vi "Hintergrund durchfuehren FT-IR.vi"() -> ()   [LabVIEW 2020, in "Linearisierung v2.lvlib"]
uses:
  Linearisierung v2.lvlib
  Visualisierungs Elemente/Button.ctl
  Visualisierungs Elemente/Zahlen-Ausgabefeld.ctl
  Visualisierungs Elemente/String - Ausgabefeld.ctl
  Seiten/FT-IR/Aktionen FT-IR Kalibrieren.ctl
  Stoerungen/Stoerungen Messgeraet/Aktionen Kommunikation Stoerung.ctl
  Sprachverwaltung/FGV Aktion Tabelle zerlegen.ctl
  Messdaten/Aktionen FGV Messdaten.ctl
  Seiten/FT-IR/FGV FT-IR Gasliste Aktionen.ctl
  Funktionstasten/Freigabe Aktionen.ctl
  Auto Kalibrieren/Aktionen Zeitstempel speichern.ctl
  Funktionstasten/Funktionstasten-Aktion.ctl
  Funktionstasten/Zustaende.ctl
  SysLog/SysLog Interface.ctl
  Seiten/FT-IR/ReadLabFile/Aktionen Lab File.ctl
  Bildwechsel/Bild-Auswahl.ctl
  Gasteiler/Aktionen FGV Gasteiler Daten.ctl
  Gasteiler/AK-Komm Gasteiler/Aktionen AK Komm.ctl
  Gasteiler/Horiba/Aktion Befehl.ctl
  Gasteiler/AK-Komm Gasteiler/Alter Gasteiler/Aktionen AK Komm_ALT.ctl
  Allgemein/allgemeine Sub-VIs.lvlib
  Seiten/FT-IR/FT-IR.lvlib
  Funktionstasten/Funktionstasten.lvlib
  Messdaten/Messdaten.lvlib
  Stoerungen/Stoerungen.lvlib
  Seiten/Erweiterte Konfig/Konfig CG-Check/CG-Check Konfig.lvlib
  Seiten/FT-IR/ReadLabFile/Read Lab File.lvlib
  Seiten/System Einstellungen V2/System Einstellungen V2.lvlib
  Seiten/System Einstellungen V2/Aktioen FGV System.ctl
  Bildwechsel/Bildwechsel.lvlib
  Sprachverwaltung/Sprachverwaltung.lvlib
  SysLog/SysLog.lvlib
  Gasteiler/AK-Komm Gasteiler/AK Komm Gasteiler.lvlib
  Gasteiler/Horiba/Horiba GDC.lvlib
  Gasteiler/AK-Komm Gasteiler/Alter Gasteiler/Alter Gasteiler.lvlib
  Gasteiler/Gasteiler.lvlib
  Auto Kalibrieren/Auto Kalibrieren.lvlib
  Gasteiler/HovaCAL_Interface/Kommunikation/Kommunikation.lvlib
panel:
  out "Konzentration CO2":T1 format="%.2f"
  out "Titelzeile":string
  out "Status":T2
  out "Konzentration H2O":T1 format="%.2f"
  in  "STARTEN":T3
  in  "ABBRECHEN":T3
  # "H2O:"
  # "CO2:"
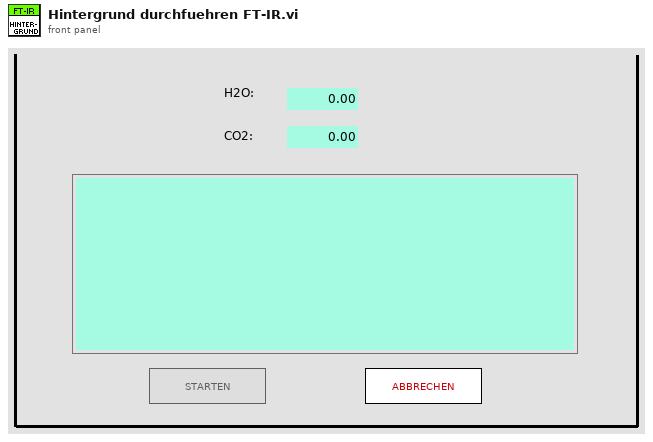
[diagram p1: front panel]
types:
  T1 = typedef "Zahlen-Ausgabefeld.ctl" = sgl
  T2 = typedef "String - Ausgabefeld.ctl" = string
  T3 = typedef "Button.ctl" = bool
  T4 = typedef "FT-IR.lvlib/Aktionen FT-IR Kalibrieren.ctl" = enum16{"Initialisieren", "Anstehende Störung", "CO2, H2O - Vergleichen", "Hintergrund starten", "Hintergrund", "Hintergrund Abgeschlossen", "Fertig", "Beenden"}
  T5 = typedef "Sprachverwaltung.lvlib/FGV Aktion Tabelle zerlegen.ctl" = enum16{"laden", "vereinzeln", "speichern"}
  T6 = typedef "Stoerungen.lvlib/Aktionen Kommunikation Stoerung.ctl" = enum16{"lesen", "init", "FT-IR Komm", "FT-IR Betriebsart", "FT-IR Hintergrund", "cRIO Komm", "PNS Komm", "Dichtheitstest", "Life Bit", "FTIR Komm AK", "PMA Komm", "FID Komm", "PMA Cal", "FID Ch4 Cal", "FID THC Cal", "Cal Timeout", "VFS 1 Komm", "VFS 2 Komm", "VFS 3 Komm", "VFS 4 Komm", "TRE 08 Komm", "CG-Test vorzeitig", "CG-Test Span 1", "CG-Test Span 2", "CG-Test Span 3", "CG-Test Messgas", "CG-Test löschen", "Test", "Amium AK", "AK Recept konfig", "AK Name konfig", "AK EKFG konfig"}
  T7 = typedef "Funktionstasten.lvlib/Freigabe Aktionen.ctl" = enum16{"prüfen", "Freigabe?", "lesen"}
  T8 = typedef "FT-IR.lvlib/FGV FT-IR Gasliste Aktionen.ctl" = enum16{"lesen", "Gasliste FT-IR", "Gasliste ausgelesen", "laden", "speichern", "löschen"}
  T9 = typedef "Messdaten.lvlib/Aktionen FGV Messdaten.ctl" = enum16{"lesen", "schreiben", "löschen", "Mittelwerte", "Komponente"}
  T10 = enum8{"Enabled", "Disabled", "Disabled and Grayed Out"}
  T11 = typedef "Auto Kalibrieren.lvlib/Aktionen Zeitstempel speichern.ctl" = enum16{"lesen", "Zeitstempel NEU", "laden", "speichern"}
  T12 = typedef "Stoerungen.lvlib/Stoerungen Messgeraete.ctl" = cluster{"FT-IR Komm":bool, "FT-IR Betriebsart":bool, "FT-IR Hintergrundscan":bool, "Dichtheitstest":bool, "cRIO Komm":bool, "PNS Komm":bool, "Life Bit":bool, "FT-IR AK Komm":bool, "PMA Komm":bool, "FID Komm":bool, "PMA Cal":bool, "FID CH4 Cal":bool, "FID THC Cal":bool, "Cal Timeout":bool, "VFS 1 Komm":bool, "VFS 2 Komm":bool, "VFS 3 Komm":bool, "VFS 4 Komm":bool, "TRE 08 Komm":bool, "CG-Test":bool, "CG-Test 1":bool, "CG-Test 2":bool, "CG-Test 3":bool, "Messgas - Eingang":bool, "Amium AK Komm":bool, "AK Rezept nicht konfiguriert ":bool, "AK Name nicht konfiguriert":bool, "AK EKFG nicht konfiguriert":bool}
  T13 = typedef "Funktionstasten.lvlib/Zustaende.ctl" = enum16{"Standby", "Pause", "Eco", "Messen", "Kalibrieren", "Spülen Filter", "Spülen Leitung", "Umgebungsluft", "0-Gas", "Cal-Gas", "CG zu PNS", "-------------", "Init 1", "Init 2", "Init 3", "Init 4", "Messen vorbereiten", "Messen durchführen", "Exit"}
  T14 = typedef "Funktionstasten.lvlib/Funktionstasten-Aktion.ctl" = enum16{"Initialisieren", "Zustand setzen", "Taste gedrückt", "Fehler speichern", "Lesen", "Manuell", "Remote", "Bitparallel", "Samplepoint", "Zeit Prüfen", "reset Umschalten"}
  T15 = typedef "SysLog.lvlib/SysLog Interface.ctl" = cluster{"FehlermeldungsCode":i32, "ErfolgsmeldungsCode":i32, "ParameterListenString":string, "Anzeige":bool, "SysLogIcon":enum16{"OK", "Warnung", "Fehler"}, "intern":bool}
  T16 = typedef "System Einstellungen V2.lvlib/Aktioen FGV System.ctl" = enum16{"lesen", "laden", "speichern", "Optionen schreiben", "Zeitstempel", "Reset BMP", "Reset SQP", "Wartung", "Werkseinstellung"}
  T17 = typedef "FT-IR.lvlib/Read Lab File.lvlib/Aktionen Lab File.ctl" = enum16{"lesen", "laden"}
  T18 = typedef "Bildwechsel.lvlib/Bild-Auswahl.ctl" = enum16{"lesen", "Initialisieren", "Beenden", "Grafik", "Anlagenübersicht", "Anlagengrenzwerte", "Log Konfig", "Gaszuordnung AO", "Erw. Konfiguration", "FT-IR  ", "Störmeldungen", "Störmeldepuffer", "Störmeldekonfig", "PNS Grenzwerte", "Statusübersicht", "Linearisierung", "ARN", "EPA Dichtheitstest", "FID", "PMA", "CalGas", "Lambda", "Interference", "Amium PNS", "EPA T90", "Interference N2O", "Scheduler", "Systemeinstellungen", "EPA Drift", "CAN Konfig"}
  T19 = typedef "Linearisierung v2.lvlib/Gasteiler.lvlib/Aktionen FGV Gasteiler Daten.ctl" = enum16{"lesen", "Gasteiler Daten", "Seriellen Param.", "MB-Endwert", "laden", "speichern", "Anforderung", "TCP", "Aufzeichnung Start"}
  T20 = typedef "Linearisierung v2.lvlib/Gasteiler.lvlib/AK Komm Gasteiler.lvlib/Aktionen AK Komm.ctl" = enum16{"lesen", "initialisieren", "beenden", "Status", "SMAN", "SREM", "STBY", "ASTF", "ASTZ", "SLST", "AGAT", "EGAK", "AGAK", "AKAK", "ADRU", "SKOP", "SVSA", "SVSZ", "SONO", "SAIR", "SNOX", "ANOX", "SSPL", "SRUC", "SLIN", "ALST", "ETYP", "SVIO", "LCYL", "CCYL", "DCYL", "SCYL", "GCYL", "DRGV", "DRDC"}
  T21 = typedef "Linearisierung v2.lvlib/Gasteiler.lvlib/Horiba GDC.lvlib/Aktion Befehl.ctl" = enum16{"lesen", "initialisieren", "Beenden", "Standby", "GD/CC", "Info", "Flow", "Alarm", "GD parameter", "GD point", "Durchfluss", "Spuelen1", "Spuelen1 On", "Spuelen1Off", "Spuelen2", "Ventil-Abfrage", "Reset"}
  T22 = typedef "Linearisierung v2.lvlib/Gasteiler.lvlib/AK Komm Gasteiler.lvlib/Alter Gasteiler.lvlib/Aktionen AK Komm_ALT.ctl" = enum16{"lesen", "initialisieren", "beenden", "SRES", "STBY", "SREM", "SMAN", "SLIN", "SLCH", "SLST", "SSPL", "AGAT", "ALST", "ASTZ", "ASTF", "AGAK", "EGAK"}
  T23 = typedef "System Einstellungen.lvlib/Optionen.ctl" = cluster{"Störmeldep.":bool, "Betriebszustände":bool, "LN2 Befüllung":bool, "Klimaanlage ?":bool, "AK in ppm":bool, "log Cal-Gas":bool, "log 0-Gas":bool, "log CG zu PNS":bool, "Reserve":bool, "Reserve1":bool, "PNS?":bool, "Container":bool, "Mit N2 spülen":bool, "Span Gas Auswahl":T24}
  T24 = typedef "Funktionstasten.lvlib/Spaneingang.ctl" = u16
  T25 = typedef "Linearisierung v2.lvlib/GasteilerType.ctl" = u16
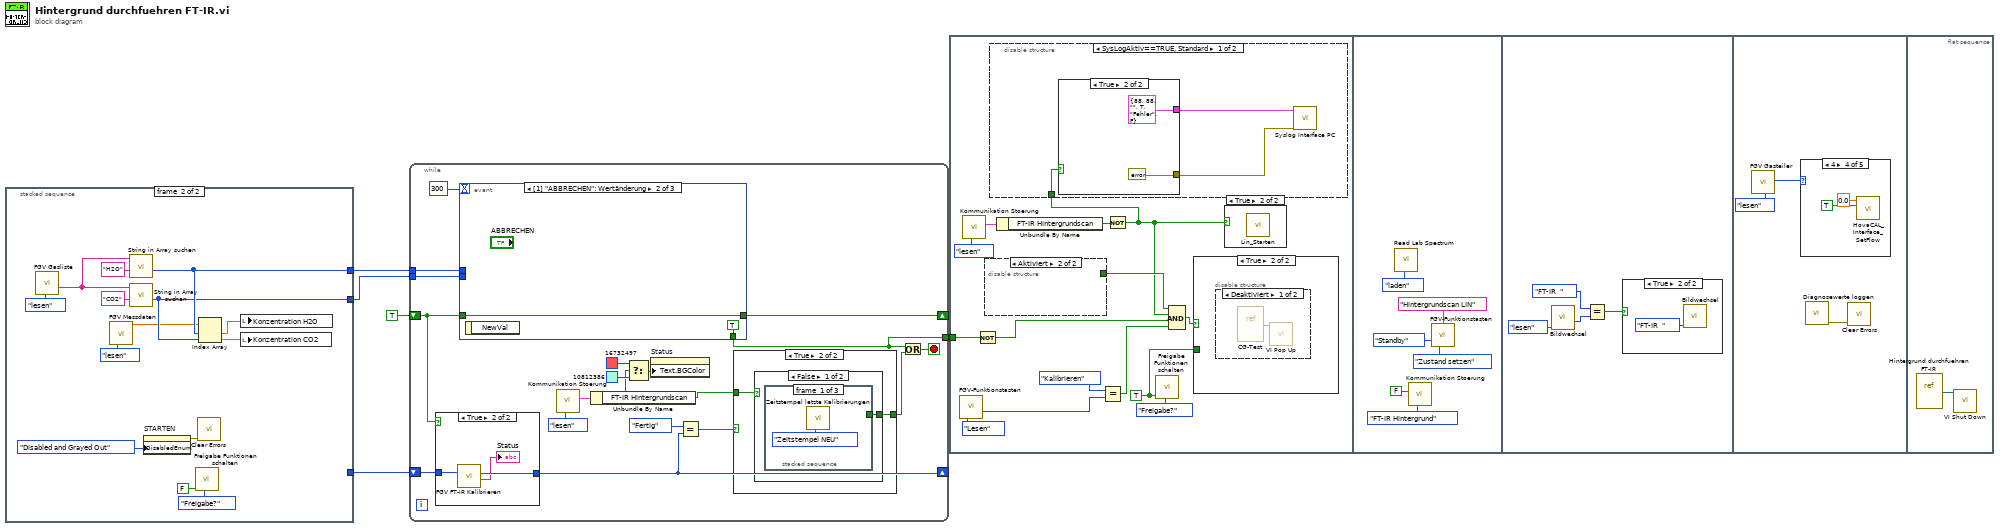
[diagram p0: block diagram]
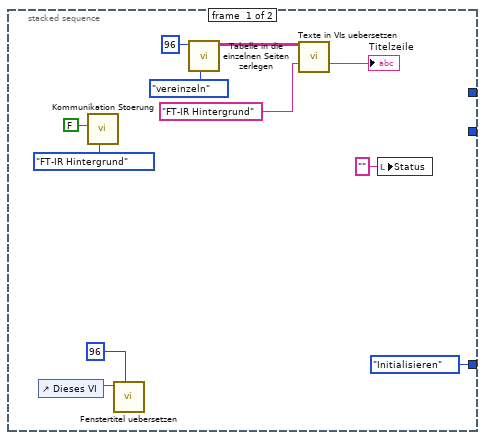
[diagram p2: hidden frame]
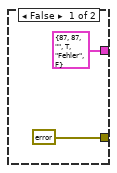
[diagram p4: hidden frame]
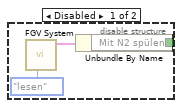
[diagram p6: hidden frame]
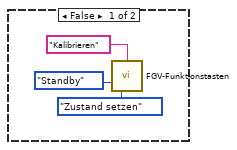
[diagram p7: hidden frame]
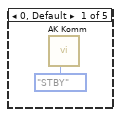
[diagram p10: hidden frame]
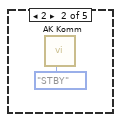
[diagram p11: hidden frame]
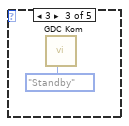
[diagram p12: hidden frame]
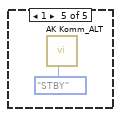
[diagram p13: hidden frame]
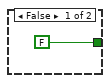
[diagram p14: hidden frame]
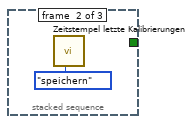
[diagram p15: hidden frame]
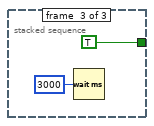
[diagram p16: hidden frame]
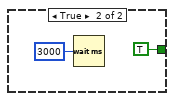
[diagram p17: hidden frame]
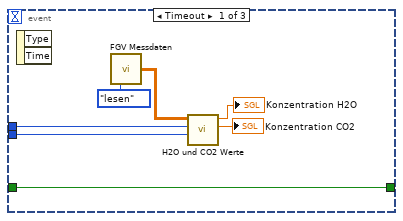
[diagram p19: hidden frame]
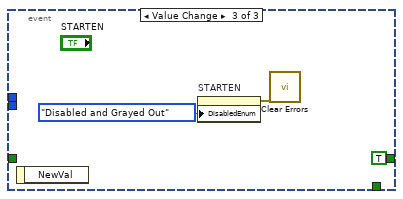
[diagram p20: hidden frame]
diagram:
  n1 = stacked-sequence {
    tunnel: [Aktionen_FT-IR_Kalibrieren."Initialisieren" ("Aktionen FT-IR Kalibrieren") _] -> w4
    tunnel: [_ w25] -> w3
    tunnel: [_ w24] -> w2
    frame #0 {
      n2 = control-ref of="Dieses VI"() -> (w7:refnum<vi>)
      n3 = call "Kommunikation Stoerung.vi"("Aktionen"=Aktionen_Kommunikation_Stoerung."FT-IR Hintergrund", "ERROR"=FALSE) -> ()  [unwired: 9 in, 1 out]
      n4 = call "Fenstertitel uebersetzen.vi"("Index (Seite)"=96, "Dieses VI"=w7) -> ()  [unwired: 6 in, 4 out]
      n5 = call "Tabelle in die einzelnen Seiten zerlegen.vi"("Aktion"=FGV_Aktion_Tabelle_zerlegen."vereinzeln", "Index (Seite)"=96) -> ("Sprachliste"=w11:string[][])  [unwired: 7 in, 2 out]
      n6 = call "Texte in VIs uebersetzen.vi"("Sprachliste"=w11, "String zum Übersetzen"="FT-IR Hintergrund") -> ("String zum Übersetzen"=→"Titelzeile":string)  [unwired: 9 in, 4 out]
      n7 = local write "Status"(T2 "" ("Status")) -> ()
    }
    frame #1 {
      n8 = call "FGV Gasliste.vi"("Aktionen"=FGV_FT-IR_Gasliste_Aktionen."lesen") -> ("Aktuelle Gasliste gesamt"=w20:T2[])  [unwired: 8 in, 2 out]
      n9 = call "FGV Messdaten.vi"("Aktionen"=Aktionen_FGV_Messdaten."lesen") -> ("Aktuelle Messwerte"=w22:sgl[])  [unwired: 6 in, 8 out]
      n10 = call "String in Array suchen.vi"("Nach String/Zeichen suchen (-)"="H2O", "String-Array"=w20) -> ("Index"=w25:i32)  [unwired: 7 in, 2 out]
      n11 = call "String in Array suchen.vi"("Nach String/Zeichen suchen (-)"="CO2", "String-Array"=w20) -> ("Index"=w24:i32)  [unwired: 7 in, 2 out]
      n12 = property on="STARTEN" class="Bool."("DisabledEnum"=T10."Disabled and Grayed Out" ("Deaktiviert")) -> (error out=w17:errorcluster)  [unwired: 2 in, 1 out]
      n13 = call "Freigabe Funktionen schalten.vi"("Aktionen"=Freigabe_Aktionen."Freigabe?", "Freigabe?"=FALSE) -> ()  [unwired: 7 in, 3 out]
      n14 = call <vilib>:"Clear Errors.vi"("error in (no error)"=w17) -> ()  [unwired: 5 in, 2 out]
      n15 = Index Array(array=w22, index #1=w25, index #2=w24) -> (element #1=w27:sgl, element #2=w26:sgl)
      n16 = local write "Konzentration H2O"(w27) -> ()
      n17 = local write "Konzentration CO2"(w26) -> ()
    }
  }
  n18 = while {
    shift-right: [w47] -> _
    shift-left: TRUE ("STARTEN") -> [w46]
    shift-right: [w42] -> _
    shift-left: w4 -> [w45]
    tunnel: w3 -> [w44]
    tunnel: w2 -> [w43]
    tunnel: [w33] -> w1
    stop <- w40 stop-if-true
    n19 = case shown="True" w46 {
      tunnel: w45 -> [w59 w62]
      tunnel: [w59 w61] -> w42
      frame False {
      }
      frame True {
        n20 = call "FGV FT-IR Kalibrieren.vi"("Aktionen FT-IR Kalibrieren"=w62) -> ("Zustand FT-IR"=→"Status":string, "Aktionen FT-IR Kalibrieren"=w61:T4)  [unwired: 9 in]
      }
    }
    n21 = event shown="[1] \"ABBRECHEN\": Wertänderung" {
      selector: _ -> [_ _ _]
      dyn-events: _ -> [_ _ _]
      timeout: 300 -> [_ _ _]
      tunnel: [_ TRUE ("ABBRECHEN") _] -> w33
      tunnel: [w69 w70 TRUE ("STARTEN")] -> w47
      tunnel: w46 -> [w69 w70 _]
      tunnel: w44 -> [w67 _ _]
      tunnel: w43 -> [w65 _ _]
      event Timeout {
        n22 = event-data() -> ()  [unwired: 1 in, 2 out]
        n23 = call "FGV Messdaten.vi"("Aktionen"=Aktionen_FGV_Messdaten."lesen") -> ("Mittelwertdaten"=w66:sgl[][])  [unwired: 6 in, 8 out]
        n24 = call "H2O und CO2 Werte.vi"("CO2 Index"=w65, "H2O Index"=w67, "Mittelwertdaten"=w66) -> ("CO2 Wert"=→"Konzentration CO2":sgl, "H2O Wert"=→"Konzentration H2O":sgl)  [unwired: 7 in]
      }
      event Value Change {
        n25 = event-data() -> ()  [unwired: 1 in, 1 out]
      }
      event Value Change {
        n26 = event-data() -> ()  [unwired: 1 in, 1 out]
        n27 = property on="STARTEN" class="Bool."("DisabledEnum"=T10."Disabled and Grayed Out" ("Deaktiviert")) -> (error out=w72:errorcluster)  [unwired: 2 in, 1 out]
        n28 = call <vilib>:"Clear Errors.vi"("error in (no error)"=w72) -> ()  [unwired: 5 in, 2 out]
      }
    }
    n29 = call "Kommunikation Stoerung.vi"("Aktionen"=Aktionen_Kommunikation_Stoerung."lesen") -> ("Störung Messgerät"=w37:T12)  [unwired: 10 in]
    n30 = Unbundle By Name(w37) -> ("FT-IR Hintergrundscan"=w31:bool)
    n31 = Select(t=u32 16732497 ("Hintergrund"), s=w31, f=u32 10812386 ("Hintergrund")) -> (s? t:f=w34:u32)
    n32 = property on="Status" class="Str (strikt)"("Text.BGColor"=w34) -> ()  [unwired: 2 in, 2 out]
    n33 = Equal?(x=Aktionen_FT-IR_Kalibrieren."Fertig", y=w42) -> (x = y?=w32:bool)
    n34 = case shown="True" w32 {
      tunnel: [FALSE w51] -> w39
      tunnel: w31 -> [_ w50]
      frame False {
      }
      frame True {
        n35 = case shown="False" w50 {
          tunnel: [w52 TRUE] -> w51
          frame False {
            n36 = stacked-sequence {
              tunnel: [_ _ TRUE] -> w52
              frame #0 {
                n37 = call "Zeitstempel letzte Kalibrierungen.vi"("Aktionen"=Aktionen_Zeitstempel_speichern."Zeitstempel NEU") -> ()  [unwired: 10 in, 1 out]
              }
              frame #1 {
                n38 = call "Zeitstempel letzte Kalibrierungen.vi"("Aktionen"=Aktionen_Zeitstempel_speichern."speichern") -> ()  [unwired: 10 in, 1 out]
              }
              frame #2 {
                n39 = Wait (ms)(milliseconds to wait=u32 3000 ("Zu wartende ms")) -> ()  [unwired: 1 out]
              }
            }
          }
          frame True {
            n40 = Wait (ms)(milliseconds to wait=u32 3000 ("Zu wartende ms")) -> ()  [unwired: 1 out]
          }
        }
      }
    }
    n41 = Or(x=w33, y=w39) -> (x .or. y?=w40:bool)
  }
  n42 = flat-sequence {
    tunnel: w1 -> [w88]
    frame #0 {
      w78 = TRUE ("Freigabe?")
      n43 = call "FGV-Funktionstasten.vi"("Aktion"=Funktionstasten-Aktion."Lesen") -> ("ausgewählte Funktion"=w83:T13)  [unwired: 7 in, 7 out]
      n44 = call "Kommunikation Stoerung.vi"("Aktionen"=Aktionen_Kommunikation_Stoerung."lesen") -> ("Störung Messgerät"=w86:T12)  [unwired: 10 in]
      n45 = Not(x=w88) -> (.not. x?=w80:bool)
      n46 = disable-structure shown="Aktiviert" {
        disable-tunnel: [w96 _] -> w77
        frame Disabled {
          n47 = call "FGV System.vi"("Aktionen"=Aktioen_FGV_System."lesen") -> ("Optionen"=w97:T23)  [unwired: 8 in, 2 out]
          n48 = Unbundle By Name(w97) -> ("Mit N2 spülen"=w96:bool)
        }
        frame Enabled {
        }
      }
      n49 = Unbundle By Name(w86) -> ("FT-IR Hintergrundscan"=w76:bool)
      n50 = Equal?(x=Zustaende."Kalibrieren", y=w83) -> (x = y?=w81:bool)
      n51 = Not(x=w76) -> (.not. x?=w75:bool)
      n52 = disable-structure shown="SysLogAktiv==TRUE, Standard" {
        disable-tunnel: w75 -> [w91 _]
        frame condition #0 (active) {
          n53 = case shown="True" w91 {
            tunnel: [errorcluster {"status"=TRUE, "code"=5558, "source"=""} ("Fehler (in)") errorcluster {"status"=FALSE, "code"=0, "source"=""} ("Fehler (in)")] -> w90
            tunnel: [T15 {"FehlermeldungsCode"=87, "ErfolgsmeldungsCode"=87, "ParameterListenString"="", "Anzeige"=TRUE, "SysLogIcon"=enum."Fehler", "intern"=FALSE} ("Cluster (in)") T15 {"FehlermeldungsCode"=88, "ErfolgsmeldungsCode"=88, "ParameterListenString"="", "Anzeige"=TRUE, "SysLogIcon"=enum."Fehler", "intern"=FALSE} ("Cluster (in)")] -> w89
            frame False {
            }
            frame True {
            }
          }
          n54 = call "Syslog Interface PC.vi"("Fehler (in)"=w90, "Cluster (in)"=w89) -> ()  [unwired: 9 in, 1 out]
        }
        frame condition #1 {
        }
      }
      n55 = call "Freigabe Funktionen schalten.vi"("Aktionen"=Freigabe_Aktionen."Freigabe?", "Freigabe?"=w78) -> ()  [unwired: 7 in, 3 out]
      n56 = Compound Arithmetic op=AND(w77, w75, w80, w81) -> (w87:bool)
      n57 = case shown="True" w87 {
        tunnel: w78 -> [_ _]
        frame False {
          n58 = call "FGV-Funktionstasten.vi"("Herkunft"="Kalibrieren", "Zustand"=Zustaende."Standby", "Aktion"=Funktionstasten-Aktion."Zustand setzen") -> ()  [unwired: 5 in, 8 out]
        }
        frame True {
          n59 = disable-structure shown="Deaktiviert" {
            frame Disabled {
              n60 = vi-ref "CG-Test.vi"() -> (w102:refnum<vi>)
              n61 = call "VI Pop Up.vi"("VI Referenz"=w102) -> ()  [unwired: 10 in, 1 out]
            }
            frame Enabled {
            }
          }
        }
      }
      n62 = case shown="True" w75 {
        frame False {
        }
        frame True {
          n63 = call "Lin_Starten.vi"() -> ()  [unwired: 11 in, 1 out]
        }
      }
    }
    frame #1 {
      n64 = call "Read Lab Spectrum.VI"("Aktionen"=Aktionen_Lab_File."laden") -> ()  [unwired: 7 in, 4 out]
      n65 = call "Kommunikation Stoerung.vi"("Aktionen"=Aktionen_Kommunikation_Stoerung."FT-IR Hintergrund", "ERROR"=FALSE) -> ()  [unwired: 9 in, 1 out]
      n66 = call "FGV-Funktionstasten.vi"("Herkunft"="Hintergrundscan LIN", "Zustand"=Zustaende."Standby", "Aktion"=Funktionstasten-Aktion."Zustand setzen") -> ()  [unwired: 5 in, 8 out]
    }
    frame #2 {
      n67 = call "Bildwechsel.vi"("nächstes Bild"=Bild-Auswahl."lesen") -> ("aktuelle Bildnummer"=w111:T18)  [unwired: 3 in, 7 out]
      n68 = Equal?(x=Bild-Auswahl."FT-IR  ", y=w111) -> (x = y?=w109:bool)
      n69 = case shown="True" w109 {
        frame False {
        }
        frame True {
          n70 = call "Bildwechsel.vi"("nächstes Bild"=Bild-Auswahl."FT-IR  ") -> ()  [unwired: 3 in, 8 out]
        }
      }
    }
    frame #3 {
      n71 = call "FGV Gasteiler.vi"("Aktionen"=Aktionen_FGV_Gasteiler_Daten."lesen") -> ("Gasteiler Type"=w116:T25)  [unwired: 11 in, 7 out]
      n72 = case shown="4" w116 {
        frame 0, Default {
          n73 = call "AK Komm.vi"("Aktionen"=Aktionen_AK_Komm."STBY") -> ()  [unwired: 4 in, 7 out]
        }
        frame 2 {
          n74 = call "AK Komm.vi"("Aktionen"=Aktionen_AK_Komm."STBY") -> ()  [unwired: 4 in, 7 out]
        }
        frame 3 {
          n75 = call "GDC Kom.vi"("Befehl"=Aktion_Befehl."Standby") -> ()  [unwired: 4 in, 7 out]
        }
        frame 4 {
          n76 = call "HovaCAL_Interface_SetFlow.vi"("sofort"=TRUE, "total flow setpoint"=0.0) -> ()  [unwired: 9 in, 1 out]
        }
        frame 1 {
          n77 = call "AK Komm_ALT.vi"("Aktionen_ALT"=Aktionen_AK_Komm_ALT."STBY") -> ()  [unwired: 6 in, 5 out]
        }
      }
      n78 = call "Diagnosewerte loggen.vi"() -> ("error out"=w114:errorcluster)  [unwired: 11 in]
      n79 = call <vilib>:"Clear Errors.vi"("error in (no error)"=w114) -> ()  [unwired: 5 in, 2 out]
    }
    frame #4 {
      n80 = vi-ref "Hintergrund durchfuehren FT-IR.vi"() -> (w123:refnum<vi>)
      n81 = call "VI Shut Down.vi"("VI Referenz"=w123) -> ()  [unwired: 11 in]
    }
  }
